vi "11713_IDN.vi"(0 "Session In":refnum<visa-resource-name>="TCPIP0::10.0.1.24::inst0::INSTR", 5 "error in":errorcluster {"code" format="%.0x"}) -> (10 "model out(str)":string, 13 "concatenated string":string, 14 "Session Out":refnum<visa-resource-name>, 19 "error out":errorcluster {"code" format="%.0x"})   [LabVIEW 2018]
panel:
  out "Address":string
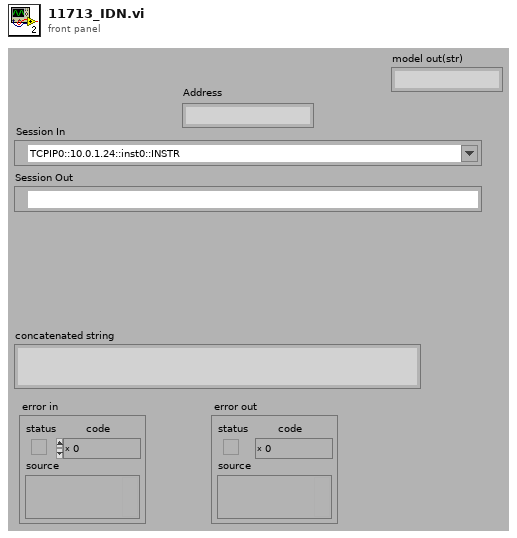
[diagram p1: front panel]
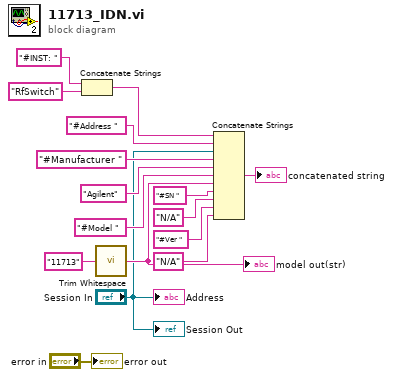
[diagram p0: block diagram]
diagram:
  n1 = Concatenate Strings("#INST: " ("string"), "RfSwitch" ("INST(name)")) -> (w4:string)
  n2 = call <vilib>:"Trim Whitespace.vi"("string"="11713" ("Model")) -> ("trimmed string"=w10:string)  [unwired: 1 in]
  "model out(str)" <- w10
  n3 = Concatenate Strings(w4, "#Address " ("string"), "Session In", "#Manufacturer ", "Agilent" ("Mfr"), "#Model ", w10, "#SN " ("string"), "N/A" ("SN"), "#Ver " ("string"), "N/A" ("Ver")) -> (→"concatenated string":string)
  "error out" <- "error in"
  "Session Out" <- "Session In"
  "Address" <- "Session In"
